vi "Meas Asynchronous Wait.vi"(5 "Allow hard kill? (True)":bool=TRUE, 7 "Wait for exit? (False)":bool, 8 "error in":errorcluster, 10 "stop button name ('btn stop')":string="btn stop", 11 "VI reference (empty)":refnum<vi>) -> (0 "error out":errorcluster, 1 "VI's error out":errorcluster, 2 "VI returned?":bool, 3 "parameter out":variant, 4 "VI exited?":bool)   [LabVIEW 2020]
doc: "This will check state of asynchronously called VI (or wait for its exit if requested). In the check only mode ('Wait for exit?' = False) it will test if the VI exited with zero timeout. If it did, it will return 'VI returned?' = True and the content of 'VI's error out' and 'parameter out' will be valid. Flag 'VI exited?' will be true whenever VI exited or VI reference is invalid.\nIn the wait mode ('Wait for exit?' = True) it will first signalize to stop by setting boolean variable named by control 'stop button name' to True (requires the SGUI library and the variable reference must be registered). Then it waits for 10s to VI exit. If it does not exit it may try to kill it (must be allowed by 'Allow hard kill?' = True). If it won't exit even after that it will return error on 'error out'. Otherwise the error out is always just a copy of input error.\nNote that this VI can return 'VI returned?' flag True only once! So when you request returned data always check the flag and if True, capture the outputs."
uses:
  varilib/varilib.lvlib
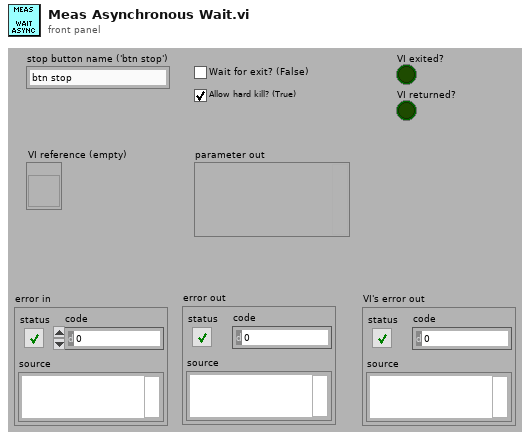
[diagram p1: front panel]
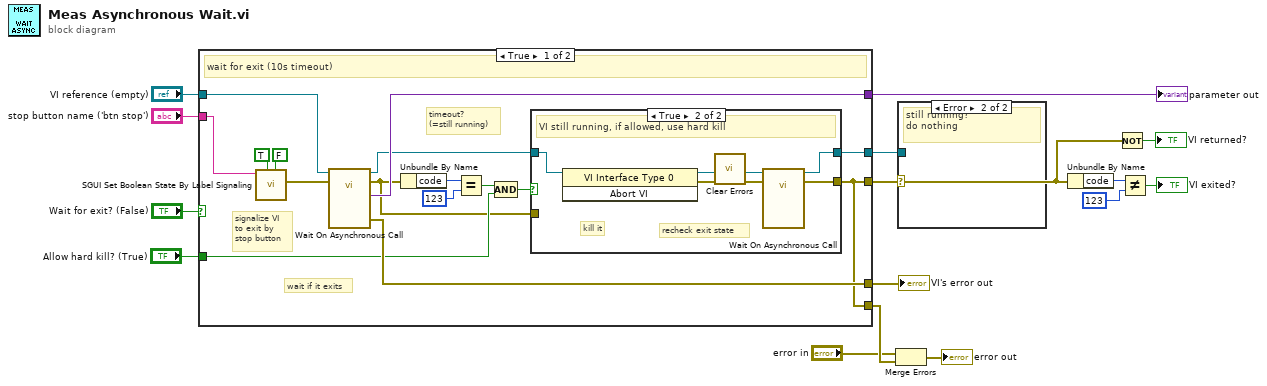
[diagram p0: block diagram]
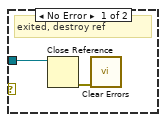
[diagram p2: hidden frame]
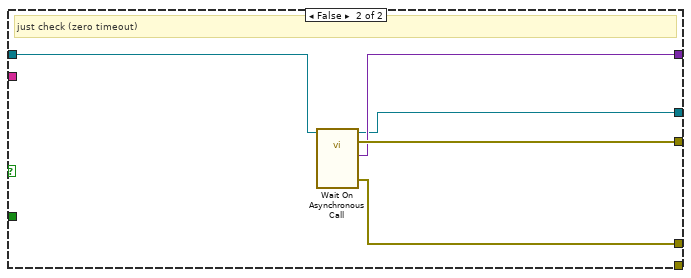
[diagram p4: hidden frame]
diagram:
  n1 = case shown="True" "Wait for exit? (False)" {
    tunnel: "VI reference (empty)" -> [w29 w44]
    tunnel: [w20 w43] -> w4
    tunnel: [w31 w42] -> w6
    tunnel: [w30 w41] -> w12
    tunnel: "stop button name ('btn stop')" -> [w16 _]
    tunnel: "Allow hard kill? (True)" -> [w23 _]
    tunnel: [w21 w40] -> w10
    tunnel: [w20 _] -> w3
    frame True {
      # "timeout?\n(=still running)"
      # "wait if it exits"
      # "signalize VI\nto exit by\nstop button"
      # "wait for exit (10s timeout)"
      n2 = call "SGUI Set Boolean State By Label Signaling.vi"("generate error if not found? (True)"=FALSE, "binary state in (False)"=TRUE, "control label(s) ('btn stop')"=w16) -> ("error out"=w19:errorcluster)  [unwired: 7 in, 1 out]
      n3 = call-by-ref "Wait On Asynchronous Call"(reference=w29, error in=w19) -> (reference out=w28:refnum<vi>, error out=w22:errorcluster, 0:"error out"=w31:errorcluster, "aux data out"=w30:variant)  [unwired: 10 in]
      n4 = Unbundle By Name(w22) -> ("code"=w27:i32)
      n5 = Equal?(x=w27, y=123) -> (x = y?=w25:bool)
      n6 = Compound Arithmetic op=AND(w25, w23) -> (w24:bool)
      n7 = case shown="True" w24 {
        tunnel: [w33 w37] -> w20
        tunnel: w28 -> [w32 w39]
        tunnel: w22 -> [w33 _]
        tunnel: [w32 w34] -> w21
        frame False {
        }
        frame True {
          # "recheck exit state"
          # "kill it"
          # "VI still running, if allowed, use hard kill"
          n8 = invoke class="VI Interface Type 0" method="Abort VI"(reference=w39) -> (reference out=w38:refnum<vi>, error out=w36:errorcluster)  [unwired: 2 in, 1 out]
          n9 = call <vilib>:"Clear Errors.vi"("error in (no error)"=w36) -> ("error out"=w35:errorcluster)  [unwired: 5 in, 1 out]
          n10 = call-by-ref "Wait On Asynchronous Call"(reference=w38, error in=w35) -> (reference out=w34:refnum<vi>, error out=w37:errorcluster)  [unwired: 10 in, 2 out]
        }
      }
    }
    frame False {
      # "just check (zero timeout)"
      n11 = call-by-ref "Wait On Asynchronous Call"(reference=w44) -> (reference out=w40:refnum<vi>, error out=w43:errorcluster, 0:"error out"=w42:errorcluster, "aux data out"=w41:variant)  [unwired: 11 in]
    }
  }
  "parameter out" <- w12
  "VI's error out" <- w6
  n12 = Merge Errors("error in", w3) -> (→"error out":errorcluster)
  n13 = case shown="Error" w4 {
    tunnel: w10 -> [w46 _]
    frame No Error {
      # "exited, destroy ref"
      n14 = Close Reference(reference=w46) -> (error out=w45:errorcluster)  [unwired: 1 in]
      n15 = call <vilib>:"Clear Errors.vi"("error in (no error)"=w45) -> ()  [unwired: 5 in, 2 out]
    }
    frame Error {
      # "still running?\ndo nothing"
    }
  }
  n16 = Unbundle By Name(w4) -> ("code"=w9:i32)
  n17 = Not(x=w4) -> (.not. x?=→"VI returned?":bool)
  n18 = Not Equal?(x=w9, y=123) -> (x != y?=→"VI exited?":bool)
